vi "IsNotNull.vi"(9 "String In":string) -> (1 "Boolean Out":bool)   [LabVIEW 2026]
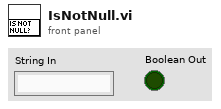
[diagram p1: front panel]
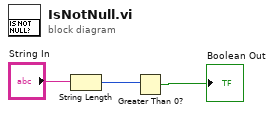
[diagram p0: block diagram]
diagram:
  n1 = String Length(string="String In") -> (length=w2:i32)
  n2 = Greater Than 0?(x=w2) -> (x > 0?=→"Boolean Out":bool)
